vi "Template Save INI Content to File.vi"(6 "Import?":bool, 7 "file":path, 8 "error in":errorcluster, 9 "key":string, 10 "section":string, 11 "refnum out":T1) -> (0 "error out":errorcluster, 3 "refnum out 2":T1)   [LabVIEW 2011]
uses:
  <vilib>/Utility/config.llb/Config Data RefNum.ctl
  <vilib>/Utility/config.llb/Read Key (String).vi
  <vilib>/Utility/config.llb/Write Key (String).vi
  <vilib>/Utility/config.llb/NI_LVConfig.lvlib
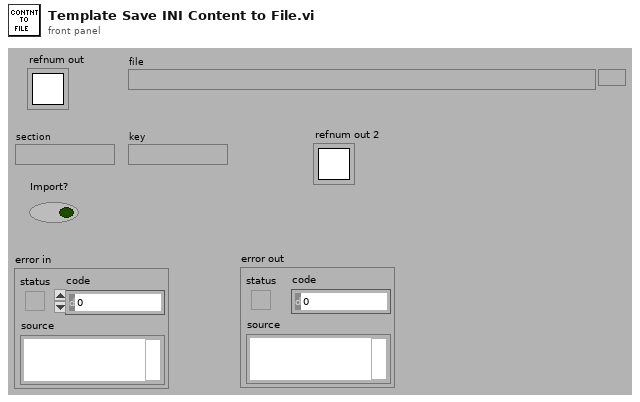
[diagram p1: front panel]
types:
  T1 = typedef "NI_LVConfig.lvlib/Config Data RefNum.ctl" = refnum<k1>
  T2 = enum16{"open", "replace", "create", "open or create", "replace or create", "replace or create with confirmation"}
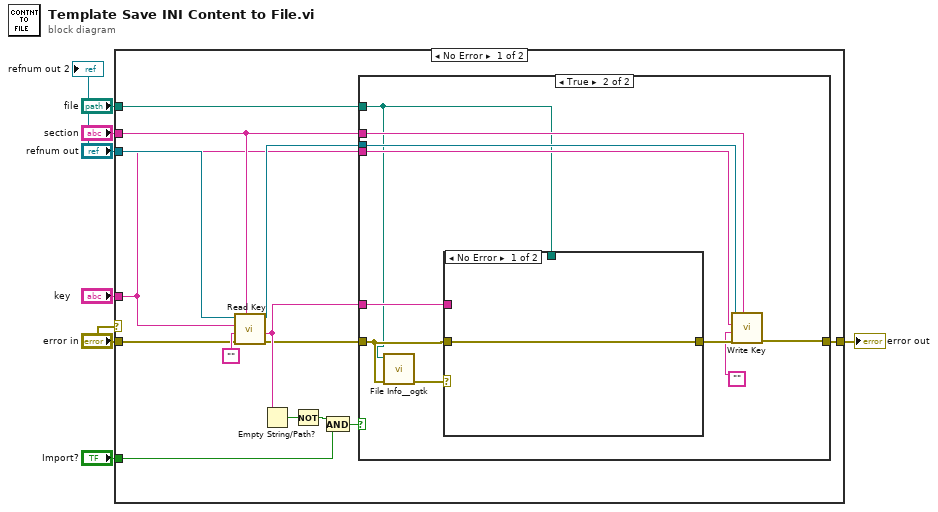
[diagram p0: block diagram]
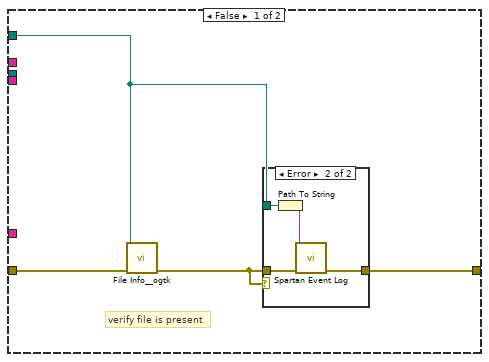
[diagram p2: hidden frame]
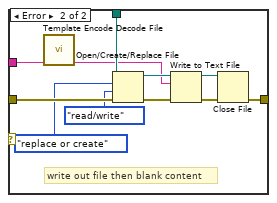
[diagram p4: hidden frame]
diagram:
  n1 = case shown="No Error" "error in" {
    tunnel: [w20 w53] -> w7
    tunnel: "file" -> [w19 _]
    tunnel: "refnum out" -> [w18 _]
    tunnel: "Import?" -> [w16 _]
    tunnel: "section" -> [w11 _]
    tunnel: "key" -> [w10 _]
    tunnel: "error in" -> [w9 w53]
    frame No Error {
      n2 = call-poly <vilib>:"Read Key.vi"("section"=w11, "error in (no error)"=w9, "default value"="", "key"=w10, "refnum"=w18) -> ("error out"=w8:errorcluster, "value"=w17:string, "refnum out"=w12:T1)  [unwired: 1 in, 3 out]
      n3 = Empty String/Path?(string/path=w17) -> (empty?=w15:bool)
      n4 = Not(x=w15) -> (.not. x?=w13:bool)
      n5 = And(x=w13, y=w16) -> (x .and. y?=w14:bool)
      n6 = case shown="True" w14 {
        tunnel: w8 -> [w25 w32]
        tunnel: [w24 w39] -> w20
        tunnel: w19 -> [w22 w31]
        tunnel: w17 -> [_ w34]
        tunnel: w12 -> [_ w38]
        tunnel: w11 -> [_ w37]
        tunnel: w10 -> [_ w36]
        frame False {
          # "verify file is present"
          n7 = call "File Info__ogtk.vi"("error in (no error)"=w25, "file"=w22) -> ("error out"=w23:errorcluster)  [unwired: 2 in, 4 out]
          n8 = case shown="Error" w23 {
            tunnel: w23 -> [w26 w30]
            tunnel: [w26 w29] -> w24
            tunnel: w22 -> [_ w28]
            frame No Error {
            }
            frame Error {
              n9 = Path To String(path=w28) -> (string=w27:string)
              n10 = call "Spartan Event Log.vi"("error in (no error)"=w30, "message (\"\")"=w27) -> ("error out"=w29:errorcluster)  [unwired: 3 in, 3 out]
            }
          }
        }
        frame True {
          n11 = call "File Info__ogtk.vi"("error in (no error)"=w32, "file"=w31) -> ("error out"=w33:errorcluster)  [unwired: 2 in, 4 out]
          n12 = case shown="No Error" w33 {
            tunnel: w32 -> [w41 w52]
            tunnel: w31 -> [_ w47]
            tunnel: [w41 w43] -> w40
            tunnel: w34 -> [_ w42]
            frame No Error {
            }
            frame Error {
              # "write out file then blank content"
              n13 = call "Template Encode Decode File.vi"("String to decode"=w42) -> ("decoded String"=w44:string)  [unwired: 10 out]
              n14 = Open/Create/Replace File(file path (use dialog)=w47, error in=w52, operation (0:open)=T2."replace or create", access (0:read/write)=enum16{"read/write", "read-only", "write-only"}."read/write") -> (refnum out=w48:refnum<file>, error out=w49:errorcluster)  [unwired: 3 out]
              n15 = Write to Text File(file (use dialog)=w48, text=w44, error in=w49) -> (refnum out=w50:refnum<file>, error out=w51:errorcluster)  [unwired: 2 out]
              n16 = Close File(refnum=w50, error in=w51) -> (error out=w43:errorcluster)  [unwired: 1 out]
            }
          }
          n17 = call-poly <vilib>:"Write Key.vi"("section"=w37, "error in (no error)"=w40, "value"="", "key"=w36, "refnum"=w38) -> ("error out"=w39:errorcluster)  [unwired: 1 in, 5 out]
        }
      }
    }
    frame Error {
    }
  }
  "error out" <- w7
  "refnum out 2" <- "refnum out"
